vi "test_blockDiagramRef.vi"   [LabVIEW 2023]
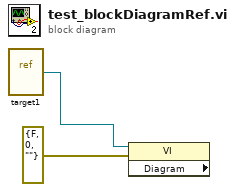
[diagram p0: block diagram]
diagram:
  n1 = vi-ref "target1.vi"() -> (w2:refnum<vi>)
  n2 = property class="VI" props=["Diagram"](reference=w2, error in=errorcluster {"status"=FALSE, "code"=0, "source"=""} ("error in (no error)")) -> ()  [unwired: 3 out]
